vi "Select emission filter.vi"(0 "Emission filter":T1, 1 "Time to wait\nafter filter change\n(ms)":u32, 2 "error in":errorcluster) -> (5 "error out":errorcluster)   [LabVIEW 2016]
uses:
  new-h-nu-ixon/Emission filters.ctl
  new-h-nu-ixon/Filter wheel settings globals.vi
  newhnu shutters/hardware status globals.vi
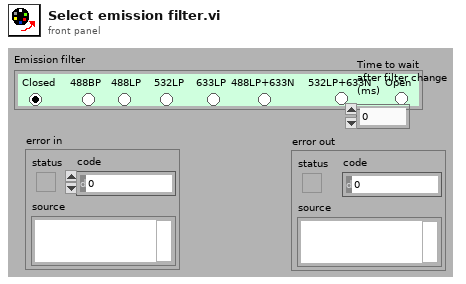
[diagram p1: front panel]
types:
  T1 = typedef "Emission filters.ctl" = enum32{" Closed ", " 488BP ", "488LP", "  532LP ", "633LP", "488LP+633N", "532LP+633N", "Open"}
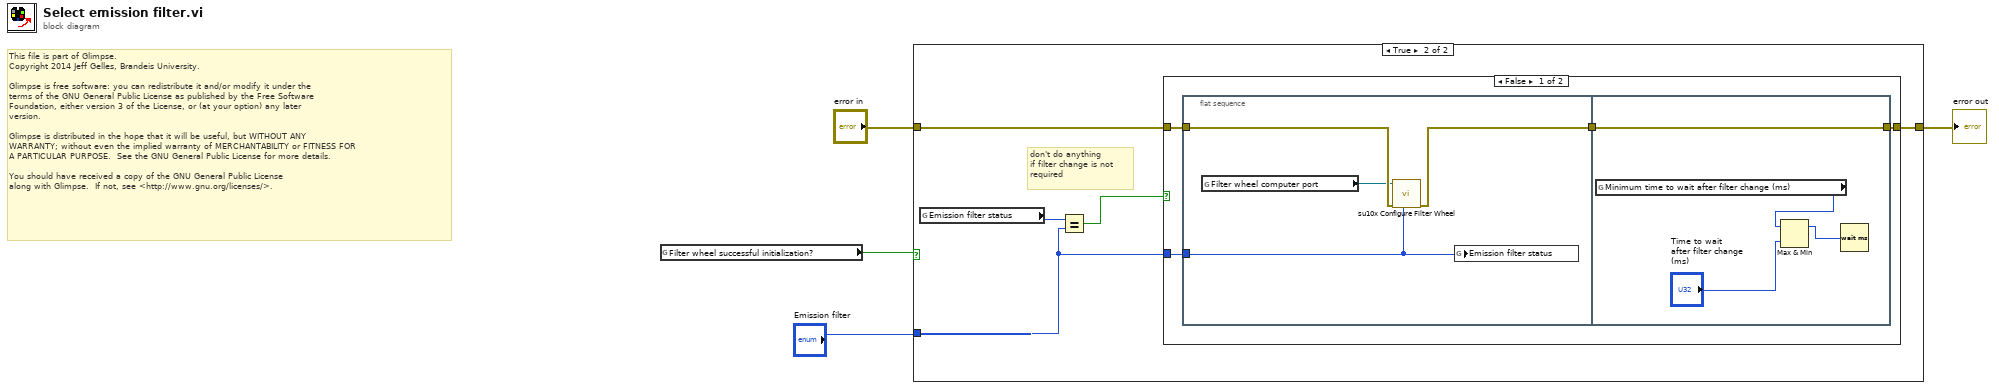
[diagram p0: block diagram]
diagram:
  # "This file is part of Glimpse. \nCopyright 2014 Jeff Gelles, Brandeis University.    \n\nGlimpse is free software: you can redistribute it and/or modify it under the \nterms of the GNU General Public License as published by the Free Software \nFoundation, either version 3 of the License, or (at your option) any later \nversion.\n\nGlimpse is distributed in the hope that it will be useful, but WITHOUT ANY \nWARRANTY; without even the implied warranty of MERCHANTABILITY or FITNESS FOR \nA PARTICULAR PURPOSE.  See the GNU General Public License for more details.\n\nYou should have received a copy of the GNU General Public License\nalong with Glimpse.  If not, see <http://www.gnu.org/licenses/>."
  n1 = global read "Filter wheel settings globals.vi" "Filter wheel successful initialization?"() -> (w4:bool)
  n2 = case shown="True" w4 {
    tunnel: [w5 w9] -> w1
    tunnel: "error in" -> [w5 w10]
    tunnel: "Emission filter" -> [_ w7]
    frame False {
    }
    frame True {
      # "don't do anything\nif filter change is not\nrequired"
      n3 = global read "hardware status globals.vi" "Emission filter status"() -> (w8:T1)
      n4 = Equal?(x=w8, y=w7) -> (x = y?=w6:bool)
      n5 = case shown="False" w6 {
        tunnel: w10 -> [w14 w23]
        tunnel: [w13 w23] -> w9
        tunnel: w7 -> [w12 _]
        frame False {
          n6 = flat-sequence {
            tunnel: w14 -> [w18]
            tunnel: w12 -> [w15]
            tunnel: [w16] -> w11
            tunnel: [w22] -> w13
            tunnel: w11 -> [w22]
            frame #0 {
              n7 = global read "Filter wheel settings globals.vi" "Filter wheel computer port"() -> (w17:refnum<visa-resource-name>)
              n8 = call <instrlib>:"su10x Configure Filter Wheel.vi"("Wheel Position (0)"=w15, "error in (no error)"=w18, "VISA resource name"=w17) -> ("error out"=w16:errorcluster)  [unwired: 2 in, 6 out]
              n9 = global write "hardware status globals.vi" "Emission filter status"(w15) -> ()
            }
            frame #1 {
              n10 = global read "Filter wheel settings globals.vi" "Minimum time to wait after filter change (ms)"() -> (w21:u32)
              n11 = Max & Min(x=w21, y="Time to wait\nafter filter change\n(ms)") -> (max(x,y)=w20:u32)  [unwired: 1 out]
              n12 = Wait (ms)(milliseconds to wait=w20) -> ()  [unwired: 1 out]
            }
          }
        }
        frame True {
        }
      }
    }
  }
  "error out" <- w1
